vi "To bytes.vi"(3 "MsgPackBool in":refnum<class "MsgPackBool.lvclass">) -> (1 "Array":u8[](array[numeric]))   [LabVIEW 2020, in "MessagePack.lvlib" / "MsgPackBool.lvclass"]
uses:
  MsgPackBool.lvclass
  MsgPackBool.lvclass/MsgPackBool.ctl
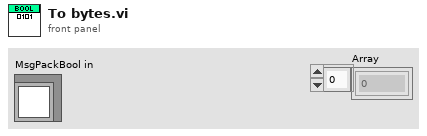
[diagram p1: front panel]
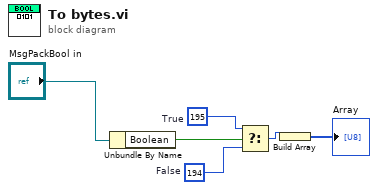
[diagram p0: block diagram]
diagram:
  w3 = u8 194  # False
  w4 = u8 195  # True
  n1 = Unbundle By Name("MsgPackBool in") -> ("Boolean"=w5:bool)
  n2 = Select(t=w4, s=w5, f=w3) -> (s? t:f=w2:u8)
  n3 = Build Array(w2) -> (→"Array":u8[])
